vi "Parameter Set.vi"(8 "error in (no error)":errorcluster, 11 "Ref In":T9={"MS SQL Connection"=refnum, "UDL File"=path "", "Time"="", "DCODE"="", "WIP+1"=0, "MC No?"=0, "POKAYOKE?"=FALSE, "Expected Result"="", "Result [Status]"="", "Clock"=0.0, "RFID"="", "WIP Queue"=refnum, "TS Parameter"={"ProfitCenterCode"="", "LineCode"="", "WorkOrderNumber"="", "Model"="", "Model_with_Prefix"="", "VendorCode"="", "SetParameterDateCode"="", "PokaYoke"=0, "Target"=1, "Live_DateCode"="", "CustomerPartNumber"="", "Hand"="", "sBarcode"=FALSE, "FCA"=0, "Ent_Stamp"=timestamp(0 s since 1904-01-01), "STS_CD"=0.0}, "Data_Queue"=[], "RFID Serial No."=""} {"TS Parameter"."FCA" format="%01d"; "TS Parameter"."Target" min=1 max=100000; "TS Parameter"."PokaYoke" min=0 max=1}) -> (0 "error out":errorcluster, 3 "Update ?":bool)   [LabVIEW 2020]
uses:
  Controls/TS_Parameter_V2.ctl
  Controls/TD SQL.ctl
  <vilib>/addons/database/Connection.llb/Conn ObjectReference.ctl
  Controls/WIP_State.ctl
  Controls/TS_Parameter.ctl
  Controls/Roting.ctl
  <menus>/Controls/Devaseelan Style/ONOFF Small.ctl
  Controls/WIP Limit.ctl
  Controls/WIP_old.ctl
  Controls/FCA CONTROL.ctl
  <vilib>/Utility/miscctls.llb/LVPointTypeDef.ctl
  MS SQL/MS_Global.vi
  <vilib>/ethernetip/ethernetip.llb/EthernetIP Tag Write DINT.vi
  <vilib>/addons/database/NI_Database_API.lvlib
  <vilib>/ethernetip/ethernetip.lvlib
panel:
  out "Origin":T1
  in  "FCA Limit":T2
  out "error out 3":errorcluster
  out "INSERT Script":string
  out "data":string[](array[string])
  out "error out 2":errorcluster
  in  "Hide":bool
  in  "User":bool
  in  "Exit":bool
  in  "Tab Control":T4(tab)
  in  "TS Parameter":T5={"ProfitCenterCode"="5603", "LineCode"="09", "WorkOrderNumber"="3534535", "Model"="29032639", "Model_with_Prefix"="0029032639", "VendorCode"="5345", "SetParameterDateCode"="04Mj", "PokaYoke"=0, "Target"=100, "Live_DateCode"="04Mj", "CustomerPartNumber"="53454353", "Hose_Type"="RH", "sBarcode"=FALSE, "FCA"=0, "Ent_Stamp"=timestamp(0 s since 1904-01-01), "STS_CD"=0.0} {"FCA" format="%01d"; "Target" min=1 max=100000; "PokaYoke" min=0 max=1}
  in  "Save":bool
  out "Date Code":string
  in  "Part Routing":T6
  in  "Line Routing":T6
  in  "Routing":bool
  in  "Part Pokayoke":T6
  in  "Line Pokayoke":T6
  in  "Pokayoke":bool
  in  "WIP Limit":T8
  in  "Save wip":bool
  in  "Finalviewing Para":bool
  in  "Hand 2":string
  out "Update":bool=TRUE
  in  "Add PKYK":bool
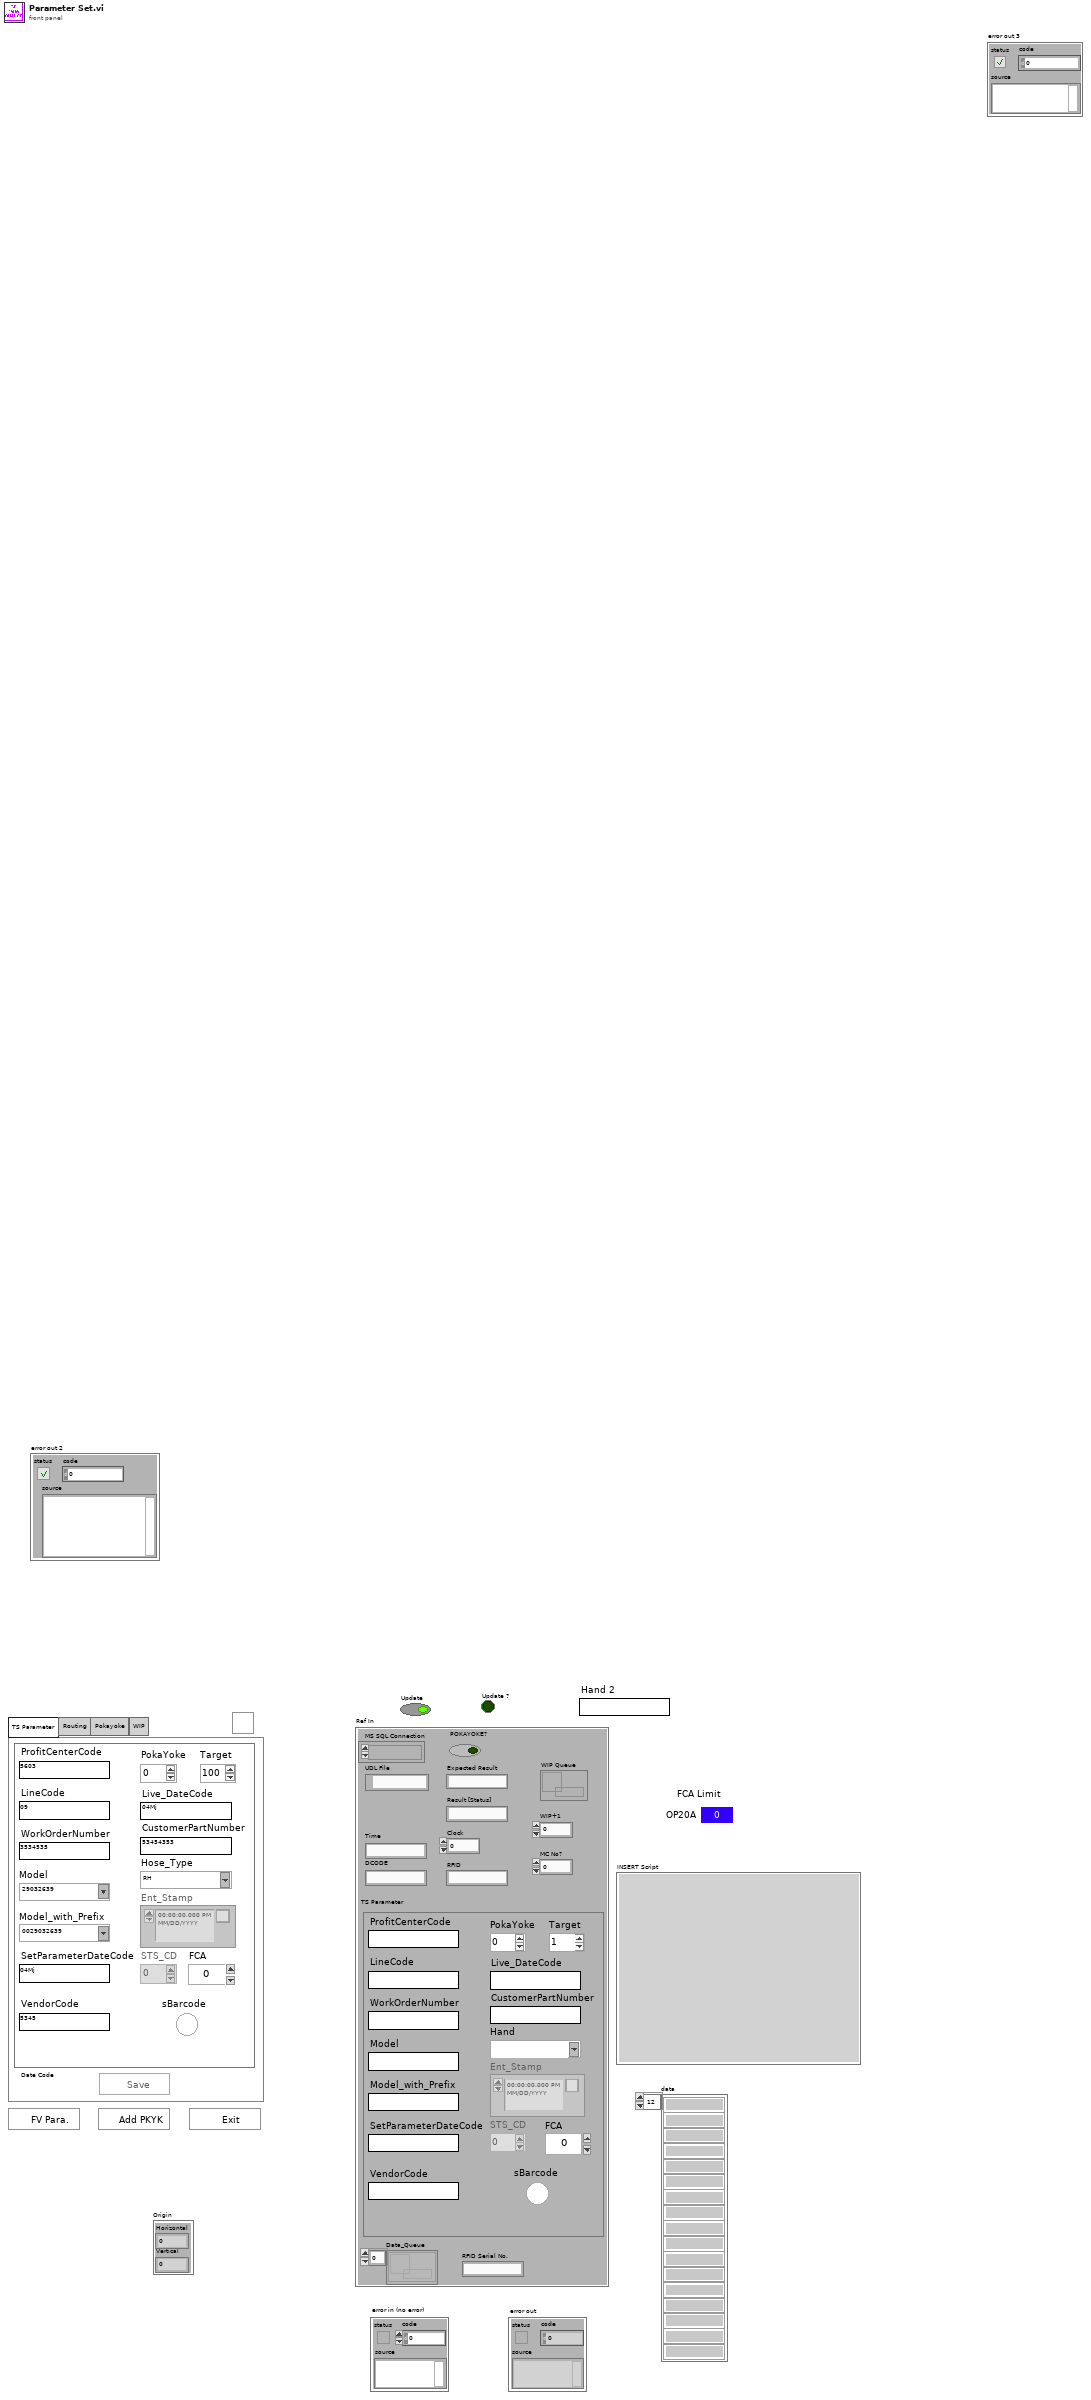
[diagram p1: front panel]
types:
  T1 = typedef "LVPointTypeDef.ctl" = cluster{"Horizontal":i16, "Vertical":i16}
  T2 = typedef "FCA CONTROL.ctl" = cluster{"OP20A":T3}
  T3 = typedef "WIP_old.ctl" = i64
  T4 = enum32{"TS Parameter", "Routing", "Pokayoke", "WIP"}
  T5 = typedef "TS_Parameter_V2.ctl" = cluster{"ProfitCenterCode":string, "LineCode":string, "WorkOrderNumber":string, "Model":string, "Model_with_Prefix":string, "VendorCode":string, "SetParameterDateCode":string, "PokaYoke":i32, "Target":i32, "Live_DateCode":string, "CustomerPartNumber":string, "Hose_Type":string, "sBarcode":bool, "FCA":i32, "Ent_Stamp":timestamp, "STS_CD":dbl}
  T6 = typedef "Roting.ctl" = cluster{"OP10":T7, "OP20A":T7, "OP20B":T7, "OP20C":T7, "OP20D":T7}
  T7 = typedef "ONOFF Small.ctl" = bool
  T8 = typedef "WIP Limit.ctl" = cluster{"OP10":T3, "OP20A":T3, "OP20B":T3, "OP20C":T3, "OP20D":T3, "OP30":T3}
  T9 = typedef "TD SQL.ctl" = cluster{"MS SQL Connection":T10, "UDL File":path, "Time":string, "DCODE":string, "WIP+1":i64, "MC No?":i32, "POKAYOKE?":bool, "Expected Result":string, "Result [Status]":string, "Clock":dbl, "RFID":string, "WIP Queue":refnum<queue>, "TS Parameter":T11, "Data_Queue":refnum<queue>[], "RFID Serial No.":string}
  T10 = typedef "NI_Database_API.lvlib/Conn ObjectReference.ctl" = refnum<k1>
  T11 = typedef "TS_Parameter.ctl" = cluster{"ProfitCenterCode":string, "LineCode":string, "WorkOrderNumber":string, "Model":string, "Model_with_Prefix":string, "VendorCode":string, "SetParameterDateCode":string, "PokaYoke":i32, "Target":i32, "Live_DateCode":string, "CustomerPartNumber":string, "Hand":string, "sBarcode":bool, "FCA":i32, "Ent_Stamp":timestamp, "STS_CD":dbl}
  T12 = enum8{"Enabled", "Disabled", "Disabled and Grayed Out"}
  T13 = typedef "LVPositionTypeDef.ctl" = cluster{"Left":i32, "Top":i32}
  T14 = cluster{"Routing[0]":bool, "Routing[1]":bool, "Routing[2]":bool, "Routing[3]":bool, "Routing[4]":bool}
  T15 = cluster{"Pokeyoke[0]":bool, "Pokeyoke[1]":bool, "Pokeyoke[2]":bool, "Pokeyoke[3]":bool, "Pokeyoke[4]":bool}
  T16 = typedef "user_log.ctl" = cluster{"eRID":u16, "eRName":string, "eRClock":string, "eRDate":timestamp, "eRLevel":string, "eRAdmin":string, "eRPassword":string}
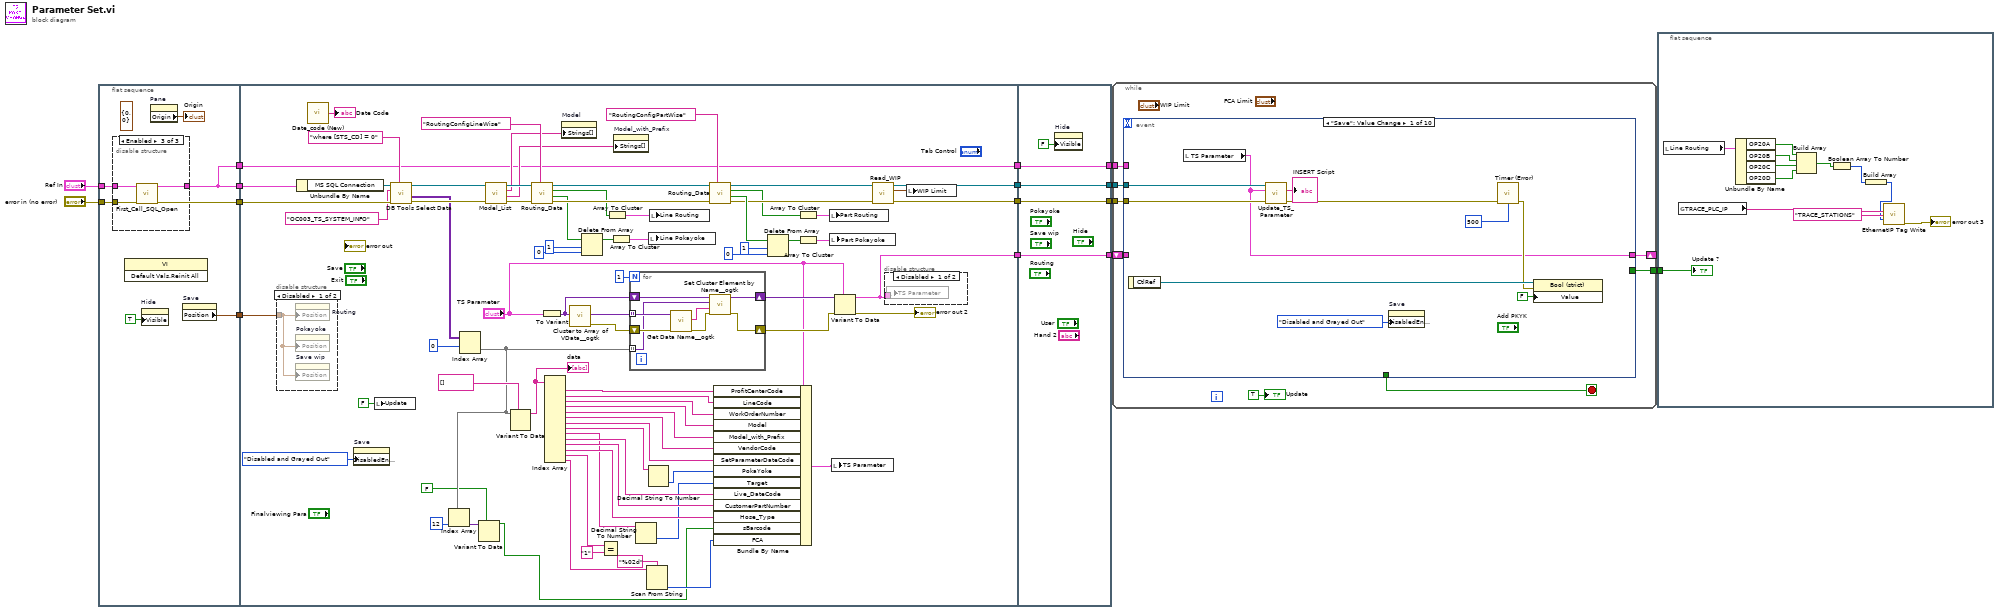
[diagram p0: block diagram]
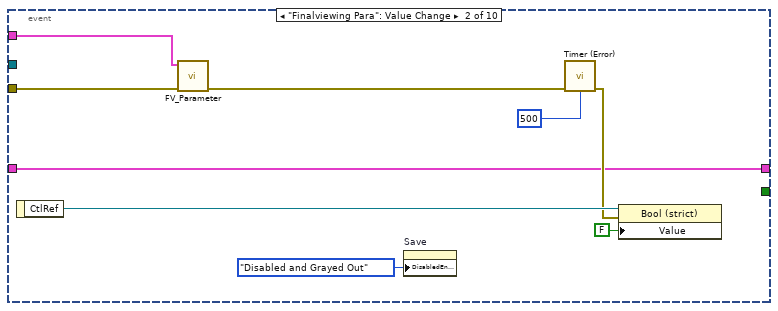
[diagram p2: hidden frame]
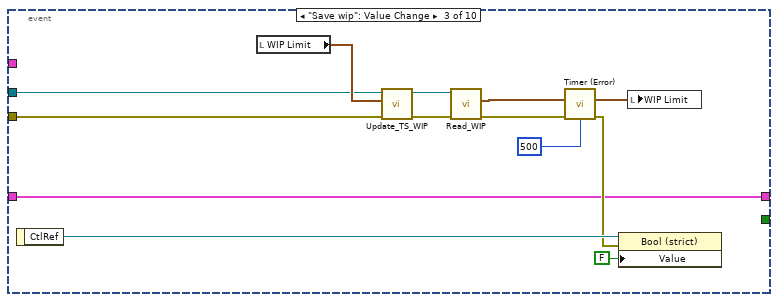
[diagram p3: hidden frame]
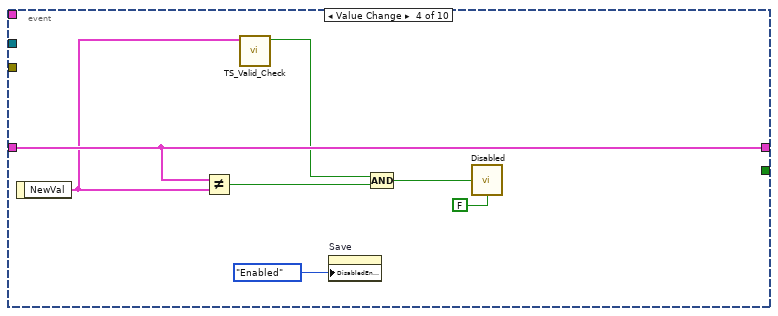
[diagram p4: hidden frame]
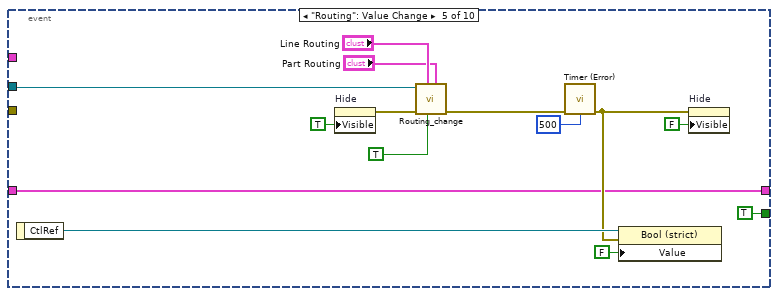
[diagram p5: hidden frame]
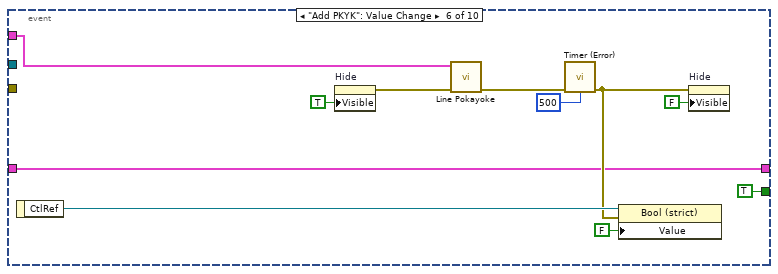
[diagram p6: hidden frame]
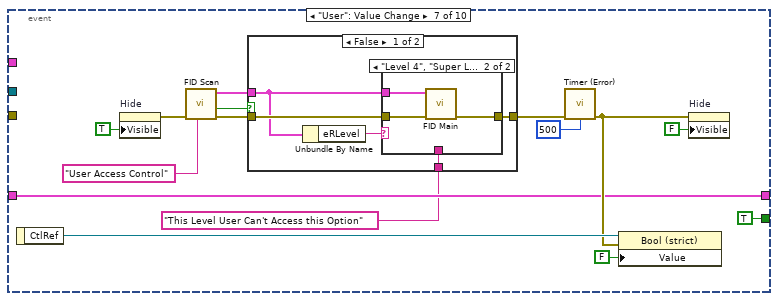
[diagram p7: hidden frame]
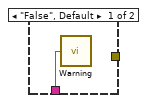
[diagram p8: hidden frame]
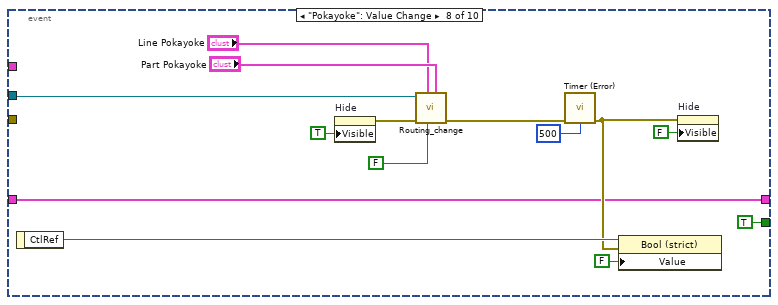
[diagram p10: hidden frame]
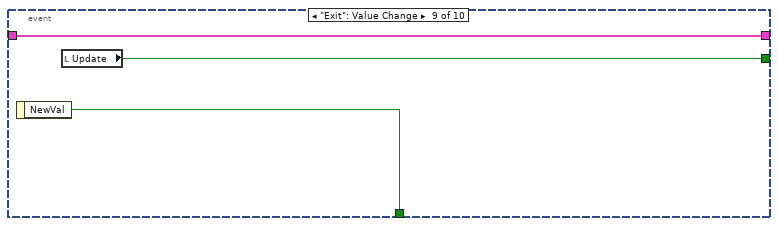
[diagram p11: hidden frame]
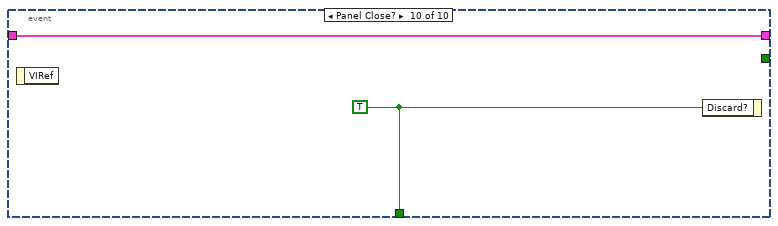
[diagram p12: hidden frame]
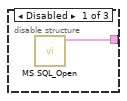
[diagram p13: hidden frame]
diagram:
  n1 = flat-sequence {
    tunnel: "error in (no error)" -> [w17]
    tunnel: "Ref In" -> [w20]
    tunnel: [w18] -> w11
    tunnel: [w17] -> w10
    tunnel: [w19] -> w4
    tunnel: [w18] -> w3
    tunnel: w11 -> [w102]
    tunnel: w10 -> [w100]
    tunnel: [w79] -> w8
    tunnel: [w81] -> w7
    tunnel: [w68] -> w5
    tunnel: w4 -> [w76]
    tunnel: w3 -> [w69]
    tunnel: [w69] -> w1
    tunnel: [w117] -> w14
    tunnel: [w118] -> w15
    tunnel: w8 -> [w118]
    tunnel: w7 -> [w117]
    tunnel: [w115] -> w6
    tunnel: w5 -> [w115]
    tunnel: [w114] -> w2
    tunnel: w1 -> [w114]
    frame #0 {
      (unwired) T1 {"Horizontal"=0, "Vertical"=0} ("Origin")
      n2 = disable-structure shown="Enabled" {
        disable-tunnel: [w22 w23 w25] -> w18
        disable-tunnel: w20 -> [_ w23 w26]
        disable-tunnel: w17 -> [_ _ w24]
        frame Disabled {
          n3 = call "MS SQL_Open.vi"() -> ("Ref Out"=w22:T9)  [unwired: 9 in, 2 out]
        }
        frame Disabled {
        }
        frame Enabled {
          n4 = call "First_Call_SQL_Open.vi"("error in (no error)"=w24, "Ref In"=w26) -> ("Ref Out"=w25:T9)  [unwired: 8 in, 1 out]
        }
      }
      n5 = invoke class="VI" method="Default Vals.Reinit All"() -> ()  [unwired: 3 in, 3 out]
      n6 = property on="Hide" class="Bool"("Visible"=TRUE) -> ()  [unwired: 2 in, 2 out]
      n7 = property on="Pane" class="Pane"() -> ("Origin"=→"Origin":T1)  [unwired: 2 in, 2 out]
      n8 = property on="Save" class="Bool (strict)"() -> ("Position"=w19:T13)  [unwired: 2 in, 2 out]
    }
    frame #1 {
      n9 = disable-structure shown="Disabled" {
        disable-tunnel: w76 -> [w105 _]
        frame Disabled {
          n10 = property on="Routing" class="Bool (strict)"("Position"=w105) -> ()  [unwired: 2 in, 2 out]
          n11 = property on="Pokayoke" class="Bool (strict)"("Position"=w105) -> ()  [unwired: 2 in, 2 out]
          n12 = property on="Save wip" class="Bool (strict)"("Position"=w105) -> ()  [unwired: 2 in, 2 out]
        }
        frame Enabled {
        }
      }
      n13 = Unbundle By Name(w102) -> ("MS SQL Connection"=w101:T10)
      n14 = call "Date_code (New).vi"() -> ("Date Code"=→"Date Code":string)  [unwired: 14 in, 1 out]
      n15 = property on="Save" class="Bool (strict)"("DisabledEnum"=T12."Disabled and Grayed Out" ("Disabled")) -> ()  [unwired: 2 in, 2 out]
      n16 = local write "Update"(FALSE ("Update")) -> ()
      n17 = call <vilib>:"DB Tools Select Data.vi"("condition"="where [STS_CD] = 0", "error in (no error)"=w100, "table"="OC003_TS_SYSTEM_INFO", "connection reference"=w101) -> ("error out"=w73:errorcluster, "data"=w64:variant[][], "connection reference out"=w75:T10)  [unwired: 2 in]
      n18 = Index Array(array=w64, index (row)=0) -> (element=w31:variant[])  [unwired: 1 in]
      n19 = Index Array(array=w31, index=12) -> (element=w29:variant)
      n20 = Variant To Data(type=FALSE ("Update"), Variant=w29) -> (data=w27:bool)  [unwired: 1 in, 1 out]
      n21 = call "Model_List.vi"("error in (no error)"=w73, "connection reference"=w75) -> ("error out"=w72:errorcluster, "Model With Prefix"=w70:string[], "Model"=w71:string[], "connection reference out"=w74:T10)  [unwired: 6 in]
      n22 = Variant To Data(type=string[] [], Variant=w31) -> (data=w56:string[])  [unwired: 1 in, 1 out]
      "data" <- w56
      n23 = call "Routing_Data.vi"("Table Name"="RoutingConfigLineWise", "error in (no error)"=w72, "Refnum in"=w74) -> ("error out"=w94:errorcluster, "Pokeyoke"=w40:bool[], "Routing"=w38:bool[], "Refnum out"=w93:T10)  [unwired: 3 in, 2 out]
      n24 = To Variant(anything="TS Parameter") -> (Variant=w59:variant)
      n25 = Index Array(array=w56) -> (element #1=w55:string, element #2=w54:string, element #3=w53:string, element #4=w52:string, element #5=w51:string, element #6=w50:string, element #7=w49:string, element #8=w44:string, element #9=w42:string, element #10=w48:string, element #11=w47:string, element #12=w46:string, element #13=w36:string, element #14=w34:string)  [unwired: 14 in]
      n26 = property on="Model" class="CmbBox"("Strings[]"=w71) -> ()  [unwired: 2 in, 2 out]
      n27 = call <userlib>:"Cluster to Array of VData__ogtk.vi"("Cluster"=w59) -> ("error out"=w63:errorcluster, "Array of VData"=w65:variant[])  [unwired: 9 in]
      n28 = Delete From Array(array=w40, length=1, index=0) -> (array with subset deleted=w89:bool[])  [unwired: 1 out]
      n29 = Equal?(x=w36, y="1") -> ()  [unwired: 1 out]
      n30 = Array To Cluster(array=w38) -> (cluster=w39:T14)
      n31 = Array To Cluster(array=w89) -> (cluster=w95:T15)
      n32 = property on="Model_with_Prefix" class="CmbBox"("Strings[]"=w70) -> ()  [unwired: 2 in, 2 out]
      n33 = for {
        N: 1 -> [_]
        tunnel: w31 -> [w108] mode=indexing
        tunnel: w65 -> [w110] mode=indexing
        shift-right: [w111] -> w61
        shift-left: w59 -> [w106]
        shift-right: [w112] -> w62
        shift-left: w63 -> [w113]
        n34 = call <userlib>:"Get Data Name__ogtk.vi"("error in (no error)"=w113, "Data"=w110) -> ("error out"=w107:errorcluster, "Data Name"=w109:string)  [unwired: 7 in, 1 out]
        n35 = call <userlib>:"Set Cluster Element by Name__ogtk.vi"("error in (no error)"=w107, "Element Name (\"\": New Element Data Name)"=w109, "New Element Value"=w108, "Cluster"=w106) -> ("error out"=w112:errorcluster, "VCluster out"=w111:variant)  [unwired: 5 in, 1 out]
      }
      n36 = Decimal String To Number(string=w42) -> (number=w41:i32)  [unwired: 2 in, 1 out]
      n37 = Scan From String(format string="%02d", input string=w34) -> (output 1=w33:i32)  [unwired: 3 in, 3 out]
      n38 = Decimal String To Number(string=w44) -> (number=w43:i32)  [unwired: 2 in, 1 out]
      n39 = local write "Line Pokayoke"(w95) -> ()
      n40 = local write "Line Routing"(w39) -> ()
      n41 = call "Routing_Data.vi"("Table Name"="RoutingConfigPartWise", "error in (no error)"=w94, "Refnum in"=w93) -> ("error out"=w80:errorcluster, "Pokeyoke"=w86:bool[], "Routing"=w37:bool[], "Refnum out"=w82:T10)  [unwired: 3 in, 2 out]
      n42 = Bundle By Name(cluster="TS Parameter", "ProfitCenterCode"=w55, "LineCode"=w54, "WorkOrderNumber"=w53, "Model"=w52, "Model_with_Prefix"=w51, "VendorCode"=w50, "SetParameterDateCode"=w49, "PokaYoke"=w43, "Target"=w41, "Live_DateCode"=w48, "CustomerPartNumber"=w47, "Hose_Type"=w46, "sBarcode"=w27, "FCA"=w33) -> (w45:T5)
      n43 = Delete From Array(array=w86, length=1, index=0) -> (array with subset deleted=w85:bool[])  [unwired: 1 out]
      n44 = Array To Cluster(array=w37) -> (cluster=w91:T14)
      n45 = Array To Cluster(array=w85) -> (cluster=w90:T15)
      n46 = local write "Part Routing"(w91) -> ()
      n47 = local write "Part Pokayoke"(w90) -> ()
      n48 = local write "TS Parameter"(w45) -> ()
      n49 = Variant To Data(error in=w62, type="TS Parameter", Variant=w61) -> (data=w68:T5, error out=→"error out 2":errorcluster)
      n50 = call "Read_WIP.vi"("error in (no error)"=w80, "Refnum in"=w82) -> ("error out"=w79:errorcluster, "WIP Limit"=w78:T8, "Refnum out"=w81:T10)  [unwired: 7 in]
      n51 = disable-structure shown="Disabled" {
        disable-tunnel: w68 -> [w104 _]
        frame Disabled {
          n52 = local write "TS Parameter"(w104) -> ()
        }
        frame Enabled {
        }
      }
      n53 = local write "WIP Limit"(w78) -> ()
    }
    frame #2 {
      n54 = property on="Hide" class="Bool"("Visible"=FALSE) -> ()  [unwired: 2 in, 2 out]
    }
  }
  n55 = while {
    tunnel: w15 -> [w125]
    tunnel: w14 -> [w124]
    tunnel: [w123] -> w9
    shift-right: [w120] -> _
    shift-left: w6 -> [w121]
    tunnel: w2 -> [w119]
    stop <- w126 stop-if-true
    n56 = event shown="[0] \"Save\": Value Change" {
      selector: _ -> [_ _ _ _ _ _ _ _ _ _]
      dyn-events: _ -> [_ _ _ _ _ _ _ _ _ _]
      timeout: _ -> [_ _ _ _ _ _ _ _ _ _]
      tunnel: [_ _ _ _ _ _ _ _ w231 w233] -> w126
      tunnel: w125 -> [w135 w139 w147 _ _ _ _ _ _ _]
      tunnel: w124 -> [w136 _ w148 _ w175 _ _ w225 _ _]
      tunnel: [_ _ _ _ TRUE ("Update") TRUE ("Update") TRUE ("Update") TRUE ("Update") w230 _] -> w123
      tunnel: w121 -> [_ w140 w146 w164 w165 w182 w197 w215 w229 w232]
      tunnel: [w130 w140 w146 w164 w165 w182 w197 w215 w229 w232] -> w120
      tunnel: w119 -> [_ w137 _ _ _ w179 _ _ _ _]
      event "Save": Value Change {
        n57 = event-data() -> ("CtlRef"=w134:refnum<vi>)  [unwired: 1 in]
        n58 = local read "TS Parameter"() -> (w130:T5)
        n59 = call "Update_TS_Parameter.vi"("error in (no error)"=w135, "TS Parameter"=w130, "Refnum in"=w136) -> ("error out"=w128:errorcluster, "INSERT Script"=→"INSERT Script":string)  [unwired: 6 in, 1 out]
        n60 = property on="Save" class="Bool (strict)"("DisabledEnum"=T12."Disabled and Grayed Out" ("Disabled")) -> ()  [unwired: 2 in, 2 out]
        n61 = call <userlib>:"Timer (Error).vi"("error in (no error)"=w128, "milliseconds to wait"=u32 500) -> ("error out"=w133:errorcluster)  [unwired: 13 in]
        n62 = property class="Bool (strict)"(reference=w134, error in=w133, "Value"=FALSE) -> ()  [unwired: 2 out]
      }
      event "Finalviewing Para": Value Change {
        n63 = event-data() -> ("CtlRef"=w145:refnum<vi>)  [unwired: 1 in]
        n64 = call "FV_Parameter.vi"("error in (no error)"=w139, "Ref in"=w137) -> ("error out"=w138:errorcluster)  [unwired: 9 in]
        n65 = property on="Save" class="Bool (strict)"("DisabledEnum"=T12."Disabled and Grayed Out" ("Disabled")) -> ()  [unwired: 2 in, 2 out]
        n66 = call <userlib>:"Timer (Error).vi"("error in (no error)"=w138, "milliseconds to wait"=u32 500) -> ("error out"=w144:errorcluster)  [unwired: 13 in]
        n67 = property class="Bool (strict)"(reference=w145, error in=w144, "Value"=FALSE) -> ()  [unwired: 2 out]
      }
      event "Save wip": Value Change {
        n68 = event-data() -> ("CtlRef"=w157:refnum<vi>)  [unwired: 1 in]
        n69 = local read "WIP Limit"() -> (w153:T8)
        n70 = call "Update_TS_WIP.vi"("error in (no error)"=w147, "WIP Limit"=w153, "Refnum in"=w148) -> ("error out"=w151:errorcluster, "Refnum out"=w152:T10)  [unwired: 7 in]
        n71 = call "Read_WIP.vi"("error in (no error)"=w151, "Refnum in"=w152) -> ("error out"=w150:errorcluster, "WIP Limit"=w149:T8)  [unwired: 7 in, 1 out]
        n72 = call <userlib>:"Timer (Error).vi"("error in (no error)"=w150, "milliseconds to wait"=u32 500) -> ("error out"=w156:errorcluster)  [unwired: 13 in]
        n73 = property class="Bool (strict)"(reference=w157, error in=w156, "Value"=FALSE) -> ()  [unwired: 2 out]
        n74 = local write "WIP Limit"(w149) -> ()
      }
      event Value Change {
        n75 = event-data() -> ("NewVal"=w161:T5)  [unwired: 1 in]
        n76 = Not Equal?(x=w164, y=w161) -> (x != y?=w163:bool)
        n77 = call "TS_Valid_Check.vi"("NewVal"=w161) -> ("Gray Out?"=w159:bool)  [unwired: 10 in]
        n78 = property on="Save" class="Bool (strict)"("DisabledEnum"=T12."Enabled" ("Disabled")) -> ()  [unwired: 2 in, 2 out]
        n79 = Compound Arithmetic op=AND(w159, w163) -> (w160:bool)
        n80 = call <userlib>:"Disabled.vi"("Enable?"=w160, "Gray Out?"=FALSE) -> ()  [unwired: 13 in, 1 out]
      }
      event "Routing": Value Change {
        n81 = event-data() -> ("CtlRef"=w178:refnum<vi>)  [unwired: 1 in]
        n82 = property on="Hide" class="Bool"("Visible"=TRUE) -> (error out=w170:errorcluster)  [unwired: 2 in, 1 out]
        n83 = call "Routing_change.vi"("Part"="Part Routing", "Routing?Pokayoke"=TRUE, "Line"="Line Routing", "error in (no error)"=w170, "Ref In"=w175) -> ("error out"=w174:errorcluster)  [unwired: 6 in]
        n84 = call <userlib>:"Timer (Error).vi"("error in (no error)"=w174, "milliseconds to wait"=u32 500) -> ("error out"=w168:errorcluster)  [unwired: 13 in]
        n85 = property class="Bool (strict)"(reference=w178, error in=w168, "Value"=FALSE) -> ()  [unwired: 2 out]
        n86 = property on="Hide" class="Bool"(error in=w168, "Visible"=FALSE) -> ()  [unwired: 1 in, 2 out]
      }
      event "Add PKYK": Value Change {
        n87 = event-data() -> ("CtlRef"=w189:refnum<vi>)  [unwired: 1 in]
        n88 = property on="Hide" class="Bool"("Visible"=TRUE) -> (error out=w181:errorcluster)  [unwired: 2 in, 1 out]
        n89 = call "Line Pokayoke.vi"("error in (no error)"=w181, "Ref In"=w179) -> ("error out"=w180:errorcluster)  [unwired: 9 in]
        n90 = call <userlib>:"Timer (Error).vi"("error in (no error)"=w180, "milliseconds to wait"=u32 500) -> ("error out"=w184:errorcluster)  [unwired: 13 in]
        n91 = property class="Bool (strict)"(reference=w189, error in=w184, "Value"=FALSE) -> ()  [unwired: 2 out]
        n92 = property on="Hide" class="Bool"(error in=w184, "Visible"=FALSE) -> ()  [unwired: 1 in, 2 out]
      }
      event "User": Value Change {
        n93 = event-data() -> ("CtlRef"=w204:refnum<vi>)  [unwired: 1 in]
        n94 = property on="Hide" class="Bool"("Visible"=TRUE) -> (error out=w195:errorcluster)  [unwired: 2 in, 1 out]
        n95 = call "FID Scan.vi"("Purpose"="User Access Control", "error in (no error)"=w195) -> ("error out"=w194:errorcluster, "Cancel ?"=w193:bool, "data"=w192:T16)  [unwired: 7 in]
        n96 = case shown="False" w193 {
          tunnel: [w209 w214] -> w196
          tunnel: w194 -> [w208 w214]
          tunnel: w192 -> [w207 _]
          tunnel: "This Level User Can't Access this Option" ("Warning in") -> [w205 _]
          frame False {
            n97 = Unbundle By Name(w207) -> ("eRLevel"=w206:string)
            n98 = case shown="\"Level 4\", \"Super Level\"" w206 {
              tunnel: [_ w213] -> w209
              tunnel: w208 -> [_ w212]
              tunnel: w207 -> [_ w211]
              tunnel: w205 -> [w210 _]
              frame "False", Default {
                n99 = call <userlib>:"Warning .vi"("Warning in"=w210) -> ()  [unwired: 15 in]
              }
              frame "Level 4", "Super Level" {
                n100 = call "FID Main.vi"("error in (no error)"=w212, "User information"=w211) -> ("error out"=w213:errorcluster)  [unwired: 9 in]
              }
            }
          }
          frame True {
          }
        }
        n101 = call <userlib>:"Timer (Error).vi"("error in (no error)"=w196, "milliseconds to wait"=u32 500) -> ("error out"=w199:errorcluster)  [unwired: 13 in]
        n102 = property class="Bool (strict)"(reference=w204, error in=w199, "Value"=FALSE) -> ()  [unwired: 2 out]
        n103 = property on="Hide" class="Bool"(error in=w199, "Visible"=FALSE) -> ()  [unwired: 1 in, 2 out]
      }
      event "Pokayoke": Value Change {
        n104 = event-data() -> ("CtlRef"=w228:refnum<vi>)  [unwired: 1 in]
        n105 = property on="Hide" class="Bool"("Visible"=TRUE) -> (error out=w222:errorcluster)  [unwired: 2 in, 1 out]
        n106 = call "Routing_change.vi"("Part"="Part Pokayoke", "Routing?Pokayoke"=FALSE, "Line"="Line Pokayoke", "error in (no error)"=w222, "Ref In"=w225) -> ("error out"=w224:errorcluster)  [unwired: 6 in]
        n107 = call <userlib>:"Timer (Error).vi"("error in (no error)"=w224, "milliseconds to wait"=u32 500) -> ("error out"=w220:errorcluster)  [unwired: 13 in]
        n108 = property class="Bool (strict)"(reference=w228, error in=w220, "Value"=FALSE) -> ()  [unwired: 2 out]
        n109 = property on="Hide" class="Bool"(error in=w220, "Visible"=FALSE) -> ()  [unwired: 1 in, 2 out]
      }
      event "Exit": Value Change {
        n110 = event-data() -> ("NewVal"=w231:bool)  [unwired: 1 in]
        n111 = local read "Update"() -> (w230:bool)
      }
      event Panel Close? {
        w233 = TRUE ("Discard?")
        n112 = event-data() -> ()  [unwired: 1 in, 1 out]
        n113 = event-data("Discard?"=w233) -> ()  [unwired: 1 in, 1 out]
      }
    }
    "Update" <- TRUE ("Update")
  }
  n114 = flat-sequence {
    tunnel: w9 -> [w245]
    frame #0 {
      n115 = local read "Line Routing"() -> (w242:T6)
      n116 = global read "MS_Global.vi" "TRACE_PLC_IP"() -> (w243:string)
      n117 = Unbundle By Name(w242) -> ("OP20A"=w240:T7, "OP20B"=w239:T7, "OP20C"=w238:T7, "OP20D"=w237:T7)
      n118 = Build Array(w240, w239, w238, w237) -> (w236:T7[])
      n119 = Boolean Array To Number(Boolean array=w236) -> (number=w235:u32)
      n120 = Build Array(w235) -> (w234:u32[])
      n121 = call-poly <vilib>:"EthernetIP Tag Write.vi"("Network Path"=w243, "Tag Name"="TRACE_STATIONS", "Data"=w234) -> ("error out"=→"error out 3":errorcluster)  [unwired: 11 in, 1 out]
      "Update ?" <- w245
    }
  }
